vi "PowerSupply.vi"() -> ()   [LabVIEW 2014]
uses:
  <vilib>/Instr/_visa.llb/VISA Configure Serial Port (Instr).vi
panel:
  in  "Vset 1":dbl format="%_3f"
  in  "Iset 1":dbl min=0.0 max=2.3 format="%_3f"
  out "Vact 1":dbl
  out "Iact 1":dbl
  in  "Switch 1":bool
  in  "Input 1":refnum<visa-resource-name>="COM6"
  # "Oven Power Supply"
  # "Vertical Magnetic Coil Power Supply"
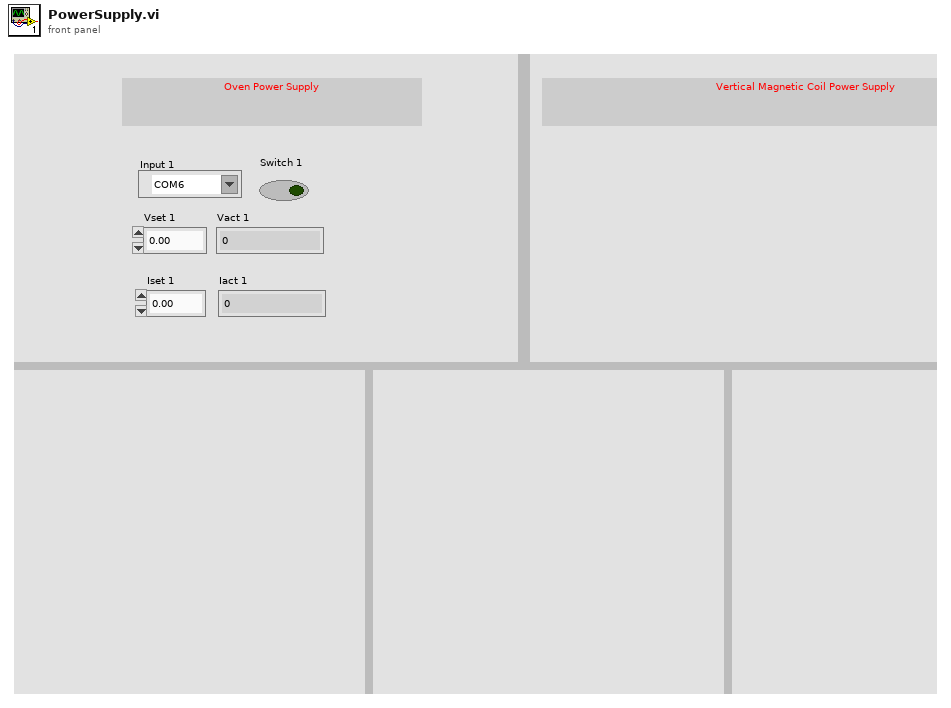
[diagram p1: front panel]
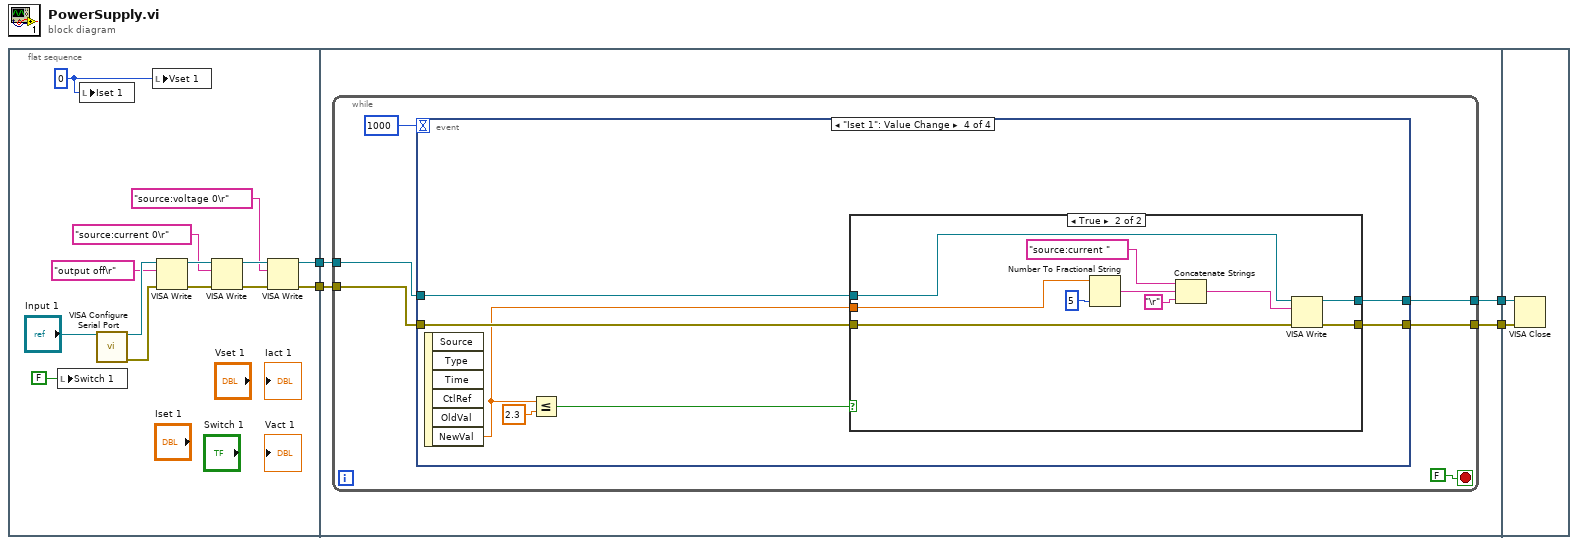
[diagram p0: block diagram]
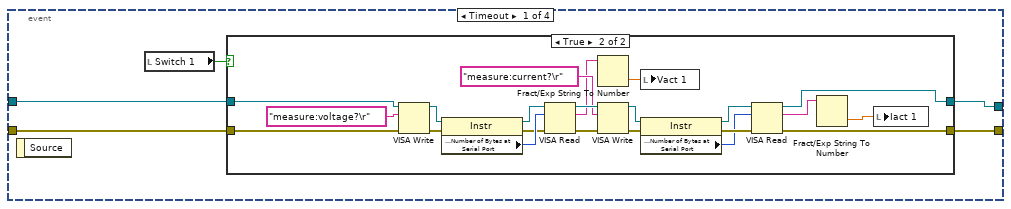
[diagram p2: hidden frame]
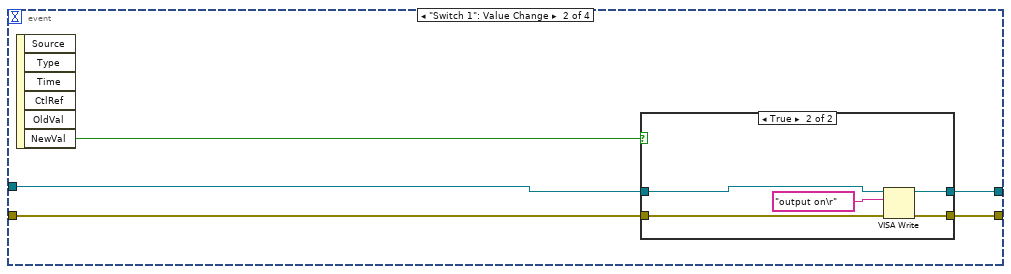
[diagram p4: hidden frame]
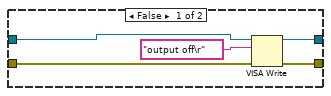
[diagram p5: hidden frame]
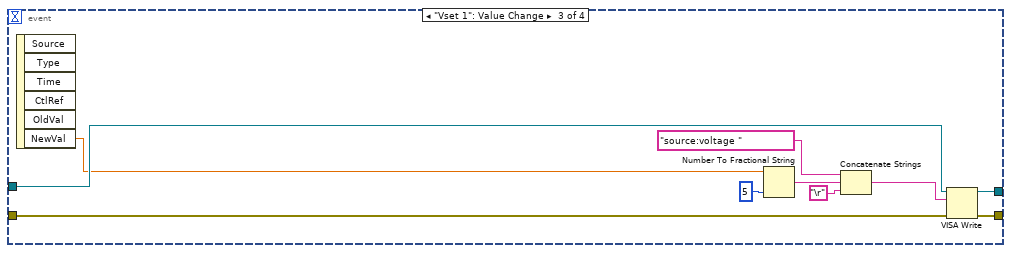
[diagram p6: hidden frame]
diagram:
  n1 = flat-sequence {
    tunnel: [w8] -> w4
    tunnel: [w7] -> w3
    tunnel: w4 -> [w22]
    tunnel: w3 -> [w21]
    tunnel: [w20] -> w2
    tunnel: [w19] -> w1
    tunnel: w2 -> [w102]
    tunnel: w1 -> [w103]
    frame #0 {
      w17 = 0
      n2 = local write "Switch 1"(FALSE) -> ()
      n3 = local write "Iset 1"(w17) -> ()
      n4 = call-poly "VISA Configure Serial Port"("VISA resource name"="Input 1") -> ("VISA resource name out"=w12:refnum<visa-resource-name>, "error out"=w11:errorcluster)  [unwired: 13 in]
      n5 = local write "Vset 1"(w17) -> ()
      n6 = VISA Write(VISA resource name=w12, write buffer="output off\r", error in (no error)=w11) -> (VISA resource name out=w14:refnum<visa-resource-name>, error out=w15:errorcluster)  [unwired: 1 out]
      n7 = VISA Write(VISA resource name=w14, write buffer="source:current 0\r", error in (no error)=w15) -> (VISA resource name out=w10:refnum<visa-resource-name>, error out=w9:errorcluster)  [unwired: 1 out]
      n8 = VISA Write(VISA resource name=w10, write buffer="source:voltage 0\r", error in (no error)=w9) -> (VISA resource name out=w8:refnum<visa-resource-name>, error out=w7:errorcluster)  [unwired: 1 out]
    }
    frame #1 {
      n9 = while {
        tunnel: w22 -> [w28]
        tunnel: w21 -> [w27]
        tunnel: [w25] -> w20
        tunnel: [w24] -> w19
        stop <- FALSE stop-if-true
        n10 = event shown="[3] \"Iset 1\": Value Change" {
          selector: _ -> [_ _ _ _]
          dyn-events: _ -> [_ _ _ _]
          timeout: 1000 -> [_ _ _ _]
          tunnel: w28 -> [w30 w59 w79 w89]
          tunnel: w27 -> [w29 w58 w78 w88]
          tunnel: [w33 w61 w74 w87] -> w25
          tunnel: [w32 w60 w73 w86] -> w24
          event Timeout {
            n11 = event-data() -> ()  [unwired: 1 in, 1 out]
            n12 = local read "Switch 1"() -> (w31:bool)
            n13 = case shown="True" w31 {
              tunnel: [w35 w39] -> w33
              tunnel: [w34 w38] -> w32
              tunnel: w30 -> [w35 w37]
              tunnel: w29 -> [w34 w36]
              frame False {
              }
              frame True {
                n14 = VISA Write(VISA resource name=w37, write buffer="measure:voltage?\r", error in (no error)=w36) -> (VISA resource name out=w56:refnum<visa-resource-name>, error out=w55:errorcluster)  [unwired: 1 out]
                n15 = property class="Instr"(reference=w56, error in=w55) -> (reference out=w54:refnum<visa-resource-name>, error out=w52:errorcluster, "Serial Settings:Number of Bytes at Serial Port"=w53:u32)
                n16 = VISA Read(VISA resource name=w54, byte count=w53, error in (no error)=w52) -> (VISA resource name out=w50:refnum<visa-resource-name>, read buffer=w40:string, error out=w48:errorcluster)  [unwired: 1 out]
                n17 = Fract/Exp String To Number(string=w40) -> (number=w51:dbl)  [unwired: 3 in, 1 out]
                n18 = VISA Write(VISA resource name=w50, write buffer="measure:current?\r", error in (no error)=w48) -> (VISA resource name out=w47:refnum<visa-resource-name>, error out=w46:errorcluster)  [unwired: 1 out]
                n19 = local write "Vact 1"(w51) -> ()
                n20 = property class="Instr"(reference=w47, error in=w46) -> (reference out=w45:refnum<visa-resource-name>, error out=w44:errorcluster, "Serial Settings:Number of Bytes at Serial Port"=w43:u32)
                n21 = VISA Read(VISA resource name=w45, byte count=w43, error in (no error)=w44) -> (VISA resource name out=w39:refnum<visa-resource-name>, read buffer=w42:string, error out=w38:errorcluster)  [unwired: 1 out]
                n22 = Fract/Exp String To Number(string=w42) -> (number=w41:dbl)  [unwired: 3 in, 1 out]
                n23 = local write "Iact 1"(w41) -> ()
              }
            }
          }
          event "Switch 1": Value Change {
            n24 = event-data() -> ("NewVal"=w62:bool)  [unwired: 1 in, 5 out]
            n25 = case shown="True" w62 {
              tunnel: w59 -> [w67 w68]
              tunnel: w58 -> [w66 w71]
              tunnel: [w64 w70] -> w61
              tunnel: [w63 w69] -> w60
              frame False {
                n26 = VISA Write(VISA resource name=w67, write buffer="output off\r", error in (no error)=w66) -> (VISA resource name out=w64:refnum<visa-resource-name>, error out=w63:errorcluster)  [unwired: 1 out]
              }
              frame True {
                n27 = VISA Write(VISA resource name=w68, write buffer="output on\r", error in (no error)=w71) -> (VISA resource name out=w70:refnum<visa-resource-name>, error out=w69:errorcluster)  [unwired: 1 out]
              }
            }
          }
          event "Vset 1": Value Change {
            n28 = event-data() -> ("NewVal"=w75:dbl)  [unwired: 1 in, 5 out]
            n29 = Number To Fractional String(number=w75, precision (6)=i16 5 ("width (-)")) -> (F-format string=w81:string)  [unwired: 2 in]
            n30 = Concatenate Strings("source:voltage ", w81, "\r") -> (w77:string)
            n31 = VISA Write(VISA resource name=w79, write buffer=w77, error in (no error)=w78) -> (VISA resource name out=w74:refnum<visa-resource-name>, error out=w73:errorcluster)  [unwired: 1 out]
          }
          event "Iset 1": Value Change {
            n32 = event-data() -> ("NewVal"=w83:dbl)  [unwired: 1 in, 5 out]
            n33 = Less Or Equal?(x=w83, y=2.3) -> (x <= y?=w84:bool)
            n34 = case shown="True" w84 {
              tunnel: w89 -> [w91 w98]
              tunnel: w88 -> [w90 w97]
              tunnel: [w91 w94] -> w87
              tunnel: [w90 w93] -> w86
              tunnel: w83 -> [_ w92]
              frame False {
              }
              frame True {
                n35 = Number To Fractional String(number=w92, precision (6)=i16 5 ("width (-)")) -> (F-format string=w100:string)  [unwired: 2 in]
                n36 = Concatenate Strings("source:current ", w100, "\r") -> (w96:string)
                n37 = VISA Write(VISA resource name=w98, write buffer=w96, error in (no error)=w97) -> (VISA resource name out=w94:refnum<visa-resource-name>, error out=w93:errorcluster)  [unwired: 1 out]
              }
            }
          }
        }
      }
    }
    frame #2 {
      n38 = VISA Close(VISA resource name=w102, error in (no error)=w103) -> ()  [unwired: 1 out]
    }
  }
